vi "feet_to_meter.vi"(1 "Feet":sgl format="%#.3f") -> (0 "Meter":sgl format="%#.3f")   [LabVIEW 2012]
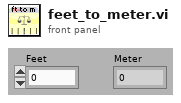
[diagram p1: front panel]
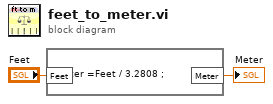
[diagram p0: block diagram]
diagram:
  n1 = formula code="Meter =Feet / 3.2808 ;"("Feet"="Feet") -> ("Meter"=→"Meter":dbl)
